vi "RSZVB Get Calibration Data Receiver Attenuation.vi"(8 "error in (no error)":errorcluster {"code" format="%.0x"}, 9 "Calibration (1)":i32=1, 10 "Channel (1)":i32=1, 11 "VISA session":refnum<visa-resource-name>) -> (0 "error out":errorcluster {"code" format="%.0x"}, 1 "Attenuation":dbl[](array[numeric]) format="%^.3e", 2 "Calibration Port":i32[](array[numeric]), 3 "dup VISA session":refnum<visa-resource-name>)   [LabVIEW 2011]
doc: "This VI queries the point delay of the channel's calibration\n\nRemote-control command(s):\n[SENSe<Ch>:]CORRection:DATA:PARameter<Cal>? RATT"
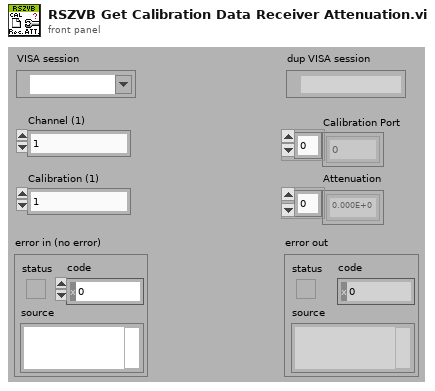
[diagram p1: front panel]
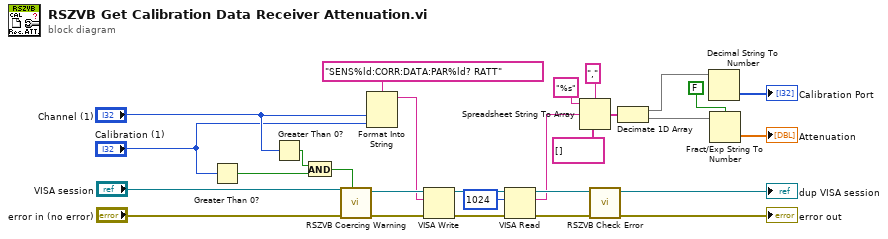
[diagram p0: block diagram]
diagram:
  n1 = Greater Than 0?(x="Calibration (1)") -> (x > 0?=w17:bool)
  n2 = Greater Than 0?(x="Channel (1)") -> (x > 0?=w18:bool)
  n3 = And(x=w18, y=w17) -> (x .and. y?=w19:bool)
  n4 = call "RSZVB Coercing Warning.vi"("In Range?"=w19, "error in (no error)"="error in (no error)", "VISA session"="VISA session") -> ("error out"=w22:errorcluster, "dup VISA session"=w23:refnum<visa-resource-name>)  [unwired: 7 in]
  n5 = Format Into String(format string="SENS%ld:CORR:DATA:PAR%ld? RATT", "Channel (1)", "Calibration (1)") -> (resulting string=w20:string)  [unwired: 2 in, 1 out]
  n6 = VISA Write(VISA resource name=w23, write buffer=w20, error in (no error)=w22) -> (VISA resource name out=w27:refnum<visa-resource-name>, error out=w28:errorcluster)  [unwired: 1 out]
  n7 = VISA Read(VISA resource name=w27, byte count=u32 1024, error in (no error)=w28) -> (VISA resource name out=w24:refnum<visa-resource-name>, read buffer=w7:string, error out=w25:errorcluster)  [unwired: 1 out]
  n8 = Spreadsheet String To Array(delimiter (Tab)=",", format string="%s", spreadsheet string=w7, array type (2D Dbl)=string[] []) -> (array=w6:string[])
  n9 = call "RSZVB Check Error.vi"("error in (no error)"=w25, "VISA session"=w24) -> ("error out"=→"error out":errorcluster, "dup VISA session"=→"dup VISA session":refnum<visa-resource-name>)  [unwired: 8 in]
  n10 = Decimate 1D Array(w6) -> (w5:string[], w2:string[])
  n11 = Decimal String To Number(string=w5) -> (number=→"Calibration Port":i32[])  [unwired: 2 in, 1 out]
  n12 = Fract/Exp String To Number(use system decimal point (T)=FALSE, string=w2) -> (number=→"Attenuation":dbl[])  [unwired: 2 in, 1 out]
